vi "DAQFIFOInit_HH.vi"(1 "error in (no error)":errorcluster) -> (0 "error out":errorcluster)   [LabVIEW 2009]
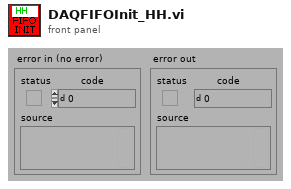
[diagram p1: front panel]
types:
  T1 = typedef "SPCConfiguration.ctt" = cluster{"SPC Initialization File":path, "Module Number":u16, "Operation Mode":u16, "Trigger Channel":tag}
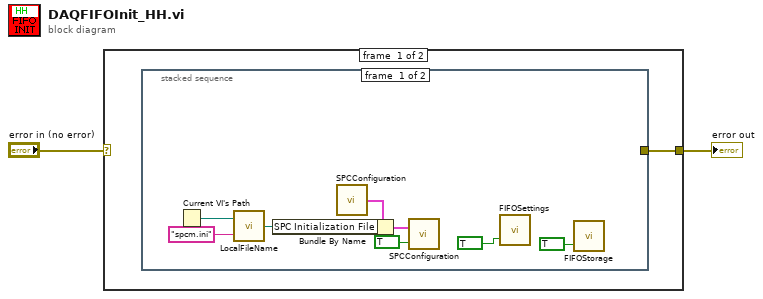
[diagram p0: block diagram]
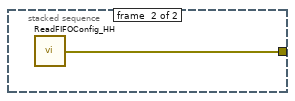
[diagram p2: hidden frame]
diagram:
  n1 = case shown="No Error" "error in (no error)" {
    selector: "error in (no error)" -> [_ w13]
    tunnel: [w3 w13] -> w1
    frame #0 {
      n2 = stacked-sequence {
        tunnel: [_ w12] -> w3
        frame #0 {
          n3 = Current VI's Path() -> (path=w7:path)
          n4 = call "LocalFileName.vi"("file name"="spcm.ini" ("name or relative path"), "VI path"=w7) -> ("full path"=w6:path)
          n5 = call "SPCConfiguration.vi"() -> ("SPC Configuration (output)"=w11:T1)  [unwired: 2 in]
          n6 = Bundle By Name(cluster=w11, "SPC Initialization File"=w6) -> (w10:T1)
          n7 = call "SPCConfiguration.vi"("Set/Get"=TRUE, "SPC Configuration (input)"=w10) -> ()  [unwired: 1 out]
          n8 = call "FIFOSettings.vi"("Set/Get"=TRUE) -> ()  [unwired: 1 in, 1 out]
          n9 = call "FIFOStorage.vi"("Set/Get"=TRUE) -> ()  [unwired: 1 in, 1 out]
        }
        frame #1 {
          n10 = call "ReadFIFOConfig_HH.vi"() -> ("error out"=w12:errorcluster)  [unwired: 1 in]
        }
      }
    }
    frame #1 {
    }
  }
  "error out" <- w1
